vi "computer_panel.vi"() -> ()   [LabVIEW 2019]
uses:
  <resource>/objmgr/ni.dex.rc
panel:
  out "error out":errorcluster
  out "Connected":bool
  out "Waveform Chart":waveform(dbl)[](graph)
  in  "stop":bool
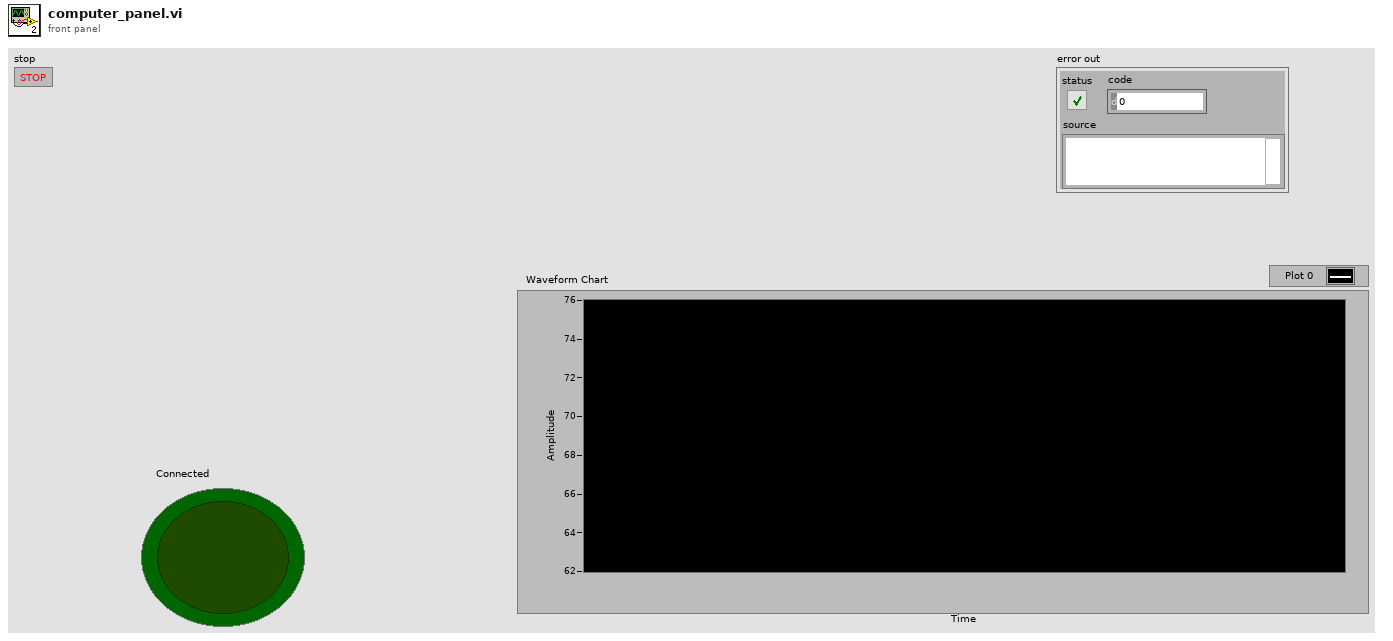
[diagram p1: front panel]
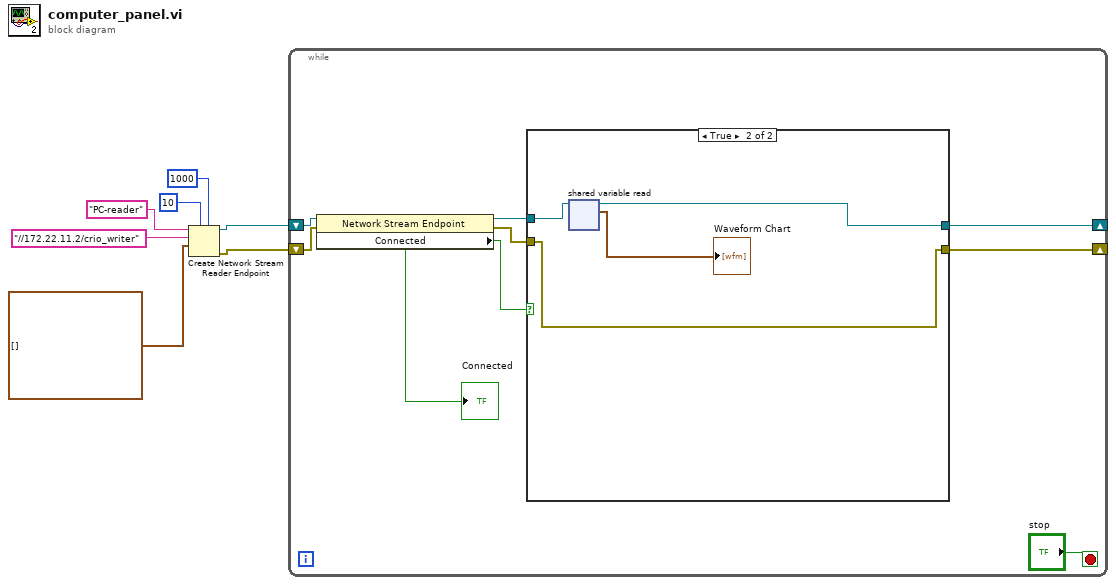
[diagram p0: block diagram]
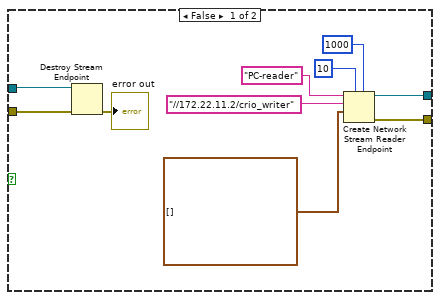
[diagram p2: hidden frame]
diagram:
  n1 = Create Network Stream Reader Endpoint(5:1000 ("timeout in ms (-1)"), 7:10 ("reader buffer size"), 9:waveform(dbl)[] [] ("data"), 10:"//172.22.11.2/crio_writer" ("writer url"), 11:"PC-reader" ("reader name")) -> (0:w2:errorcluster, 3:w3:refnum<k21>)  [unwired: 2 in]
  n2 = while {
    shift-right: [w9] -> _
    shift-left: w3 -> [w14]
    shift-right: [w8] -> _
    shift-left: w2 -> [w10]
    stop <- "stop" stop-if-true
    n3 = property class="Network Stream Endpoint"(reference=w14, error in=w10) -> (reference out=w13:refnum<k21>, error out=w11:errorcluster, "Connected"=w12:bool)
    "Connected" <- w12
    n4 = case shown="True" w12 {
      tunnel: w13 -> [w25 w29]
      tunnel: w11 -> [w24 w28]
      tunnel: [w18 w27] -> w9
      tunnel: [w17 w28] -> w8
      frame False {
        n5 = Destroy Stream Endpoint(8:w24, 11:w25) -> (0:→"error out":errorcluster)
        n6 = Create Network Stream Reader Endpoint(5:1000 ("timeout in ms (-1)"), 7:10 ("reader buffer size"), 9:waveform(dbl)[] [] ("data"), 10:"//172.22.11.2/crio_writer" ("writer url"), 11:"PC-reader" ("reader name")) -> (0:w17:errorcluster, 3:w18:refnum<k21>)  [unwired: 2 in]
      }
      frame True {
        n7 = shared-variable-read(w29) -> (w27:refnum<k21>, →"Waveform Chart":waveform(dbl)[])  [unwired: 2 in, 2 out]
      }
    }
  }
